vi "Large File - create Temperature Graph.vi"(4 "error in (no error)":errorcluster, 7 "tdms file":refnum<k34>) -> (0 "error out":errorcluster, 1 "Min and Max Temperatures":dbl[][](array[numeric]), 2 "Temperature (Degrees C) against Time (s)":waveform(dbl)(graph), 3 "tdms file out":refnum<k34>)   [LabVIEW 2015]
uses:
  <vilib>/measure/maresamp.llb/Resample Waveform (continuous).vi
  <vilib>/Waveform/WDTOps.llb/WDT Append Waveforms DBL.vi
  <vilib>/measure/NI_MAPro.lvlib
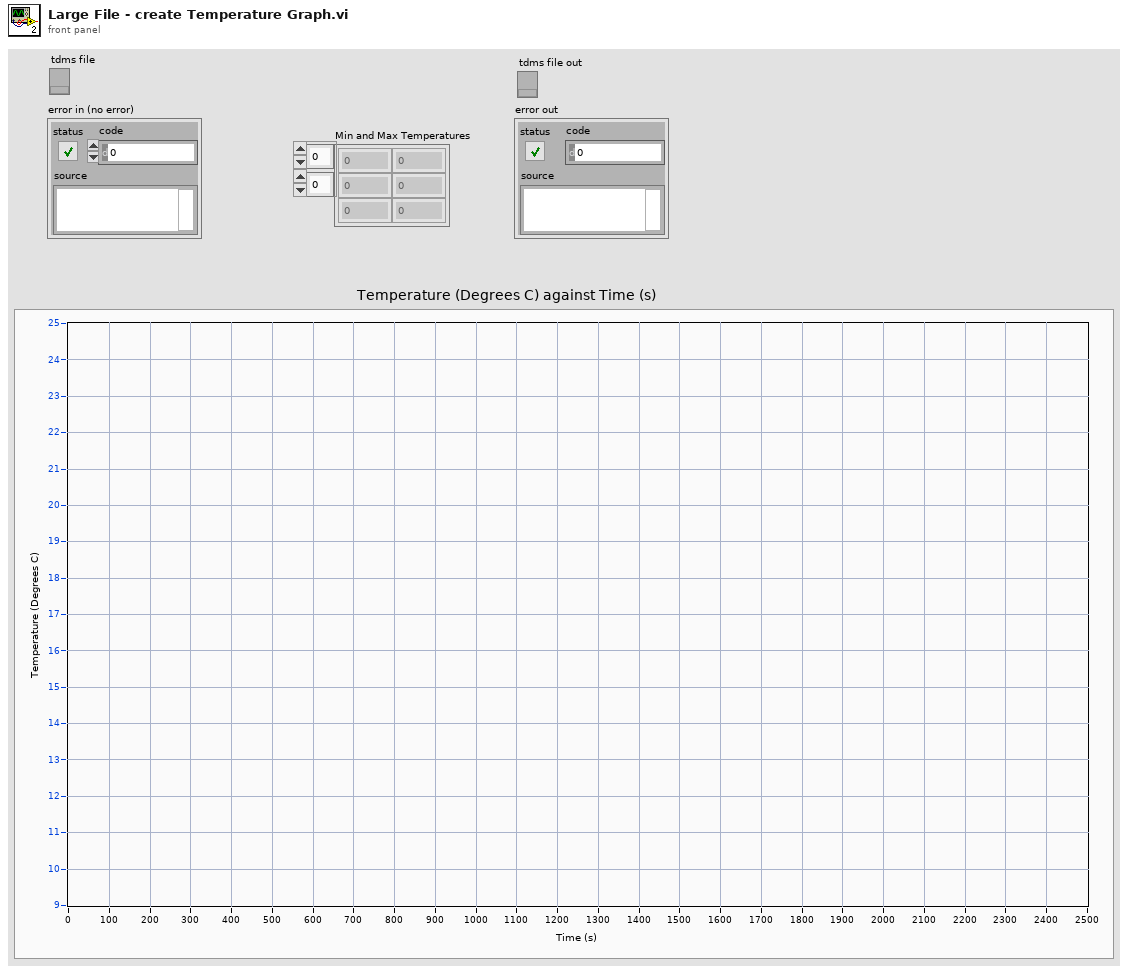
[diagram p1: front panel]
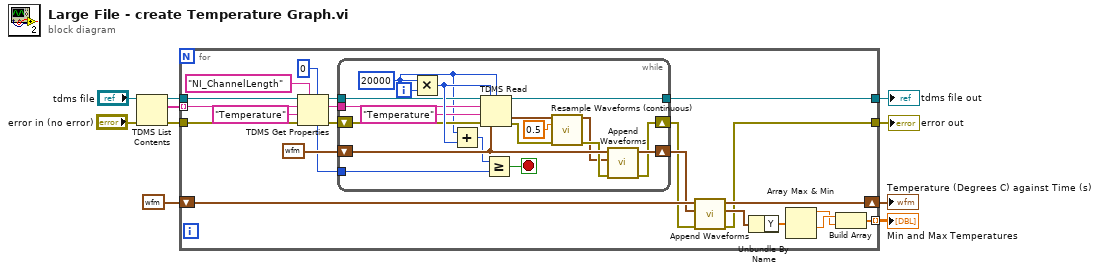
[diagram p0: block diagram]
diagram:
  n1 = TDMS List Contents(4:"error in (no error)", 7:"tdms file") -> (0:w9:errorcluster, 2:w8:string[], 3:w7:refnum<k34>)  [unwired: 1 in, 1 out]
  n2 = for {
    tunnel: w7 -> [w16]
    tunnel: w8 -> [w17] mode=indexing
    tunnel: w9 -> [w14]
    tunnel: [w31] -> w2
    tunnel: [w11] -> w1
    shift-right: [w26] -> w6
    shift-left: waveform(dbl) {"t0"=timestamp(0 s since 1904-01-01), "dt"=0.5, "Y"=[]} ("Waveform") -> [w27]
    tunnel: [w24] -> w5 mode=indexing
    n3 = TDMS Get Properties(5:0, 7:"NI_ChannelLength" ("property name"), 8:w14, 9:"Temperature" ("channel name"), 10:w17, 11:w16) -> (0:w15:errorcluster, 2:w18:string, 3:w19:refnum<k34>, 4:w13:i32)  [unwired: 2 out]
    n4 = while {
      tunnel: w18 -> [w35]
      shift-right: [w47] -> w12
      shift-left: w15 -> [w37]
      shift-right: [w48] -> w25
      shift-left: waveform(dbl) {"t0"=timestamp(0 s since 1904-01-01), "dt"=0.5, "Y"=[]} ("Waveform") -> [w49]
      tunnel: w19 -> [w36]
      tunnel: [w50] -> w31
      tunnel: w13 -> [w33]
      i -> [w41]
      stop <- w38 stop-if-true
      w32 = i64 20000
      n5 = Multiply(x=w32, y=w41) -> (x*y=w40:i64)
      n6 = Add(x=w32, y=w40) -> (x+y=w39:i64)
      n7 = TDMS Read(0:w36, 1:w40, 2:w32, 5:w35, 7:"Temperature", 11:w37, 12:w49) -> (4:w50:refnum<k34>, 10:w44:waveform(dbl), 15:w45:errorcluster)  [unwired: 1 in, 3 out]
      n8 = Greater Or Equal?(x=w39, y=w33) -> (x >= y?=w38:bool)
      n9 = call-poly <vilib>:"Resample Waveforms (continuous).vi"("waveform in"=w44, "dt"=0.5, "error in (no error)"=w45) -> ("resampled waveform out"=w42:waveform(dbl), "error out"=w43:errorcluster)  [unwired: 8 in, 3 out]
      n10 = call-poly <vilib>:"Append Waveforms.vi"("error in (no error)"=w43, "waveform B"=w42, "waveform A"=w49) -> ("error out"=w47:errorcluster, "waveform out"=w48:waveform(dbl))  [unwired: 7 in]
    }
    n11 = call-poly <vilib>:"Append Waveforms.vi"("error in (no error)"=w12, "waveform B"=w25, "waveform A"=w27) -> ("error out"=w11:errorcluster, "waveform out"=w26:waveform(dbl))  [unwired: 7 in]
    n12 = Unbundle By Name(w25) -> ("Y"=w30:dbl[])
    n13 = Array Max & Min(array=w30) -> (max value=w28:dbl, min value=w29:dbl)  [unwired: 2 out]
    n14 = Build Array(w29, w28) -> (w24:dbl[])
  }
  "Temperature (Degrees C) against Time (s)" <- w6
  "Min and Max Temperatures" <- w5
  "tdms file out" <- w2
  "error out" <- w1
